vi "Set Current Range in Sweep.vi"(0 "VISA resource name":refnum<visa-resource-name>="GPIB0::24::INSTR", 5 "R":i32, 11 "error in (no error)":errorcluster) -> (4 "VISA resource name out":refnum<visa-resource-name>="GPIB0::24::INSTR", 15 "error out":errorcluster)   [LabVIEW 2010]
uses:
  <instrlib>/Keithley 2400/Keithley 24XX.lvlib
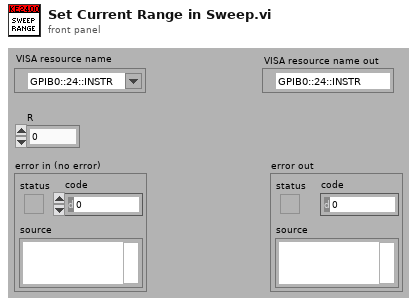
[diagram p1: front panel]
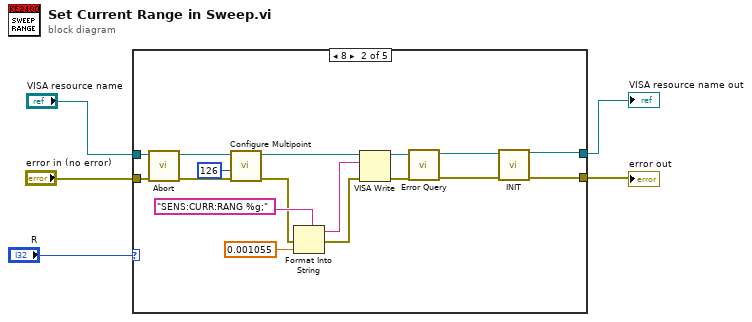
[diagram p0: block diagram]
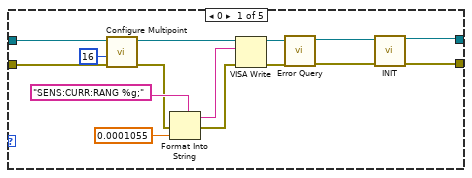
[diagram p2: hidden frame]
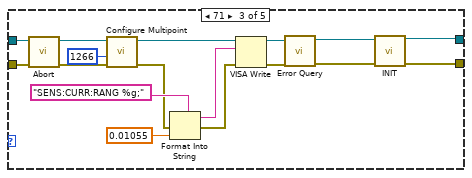
[diagram p3: hidden frame]
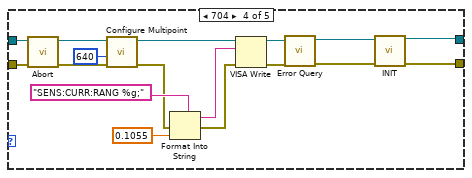
[diagram p4: hidden frame]
diagram:
  n1 = case shown="8" "R" {
    tunnel: [w15 w32 w49 w66 w73] -> w5
    tunnel: [w17 w34 w51 w68 w72] -> w4
    tunnel: "VISA resource name" -> [w10 w22 w39 w56 w73]
    tunnel: "error in (no error)" -> [w9 w27 w44 w61 w72]
    frame 0 {
      n2 = call <instrlib>:"Configure Multipoint.vi"("error in (no error)"=w9, "Trigger Count (1)"=16, "VISA resource name"=w10) -> ("error out"=w8:errorcluster, "VISA resource name out"=w7:refnum<visa-resource-name>)  [unwired: 7 in]
      n3 = Format Into String(format string="SENS:CURR:RANG %g;" ("Manual Range"), error in=w8, 0.0001055 ("R 2")) -> (resulting string=w12:string, error out=w11:errorcluster)  [unwired: 1 in]
      n4 = VISA Write(VISA resource name=w7, write buffer=w12, error in (no error)=w11) -> (VISA resource name out=w19:refnum<visa-resource-name>, error out=w18:errorcluster)  [unwired: 1 out]
      n5 = call <instrlib>:"Error Query.vi"("error in (no error)"=w18, "VISA resource name"=w19) -> ("error out"=w20:errorcluster, "VISA resource name out"=w16:refnum<visa-resource-name>)  [unwired: 6 in, 2 out]
      n6 = call "INIT.vi"("VISA resource name"=w16, "error in (no error)"=w20) -> ("VISA resource name out"=w15:refnum<visa-resource-name>, "error out"=w17:errorcluster)  [unwired: 12 in]
    }
    frame 8 {
      n7 = call <instrlib>:"Abort.vi"("error in (no error)"=w27, "VISA resource name"=w22) -> ("error out"=w23:errorcluster, "VISA resource name out"=w21:refnum<visa-resource-name>)  [unwired: 8 in]
      n8 = call <instrlib>:"Configure Multipoint.vi"("error in (no error)"=w23, "Trigger Count (1)"=126, "VISA resource name"=w21) -> ("error out"=w26:errorcluster, "VISA resource name out"=w25:refnum<visa-resource-name>)  [unwired: 7 in]
      n9 = Format Into String(format string="SENS:CURR:RANG %g;" ("Manual Range"), error in=w26, 0.001055 ("R 2")) -> (resulting string=w29:string, error out=w28:errorcluster)  [unwired: 1 in]
      n10 = VISA Write(VISA resource name=w25, write buffer=w29, error in (no error)=w28) -> (VISA resource name out=w36:refnum<visa-resource-name>, error out=w35:errorcluster)  [unwired: 1 out]
      n11 = call <instrlib>:"Error Query.vi"("error in (no error)"=w35, "VISA resource name"=w36) -> ("error out"=w37:errorcluster, "VISA resource name out"=w33:refnum<visa-resource-name>)  [unwired: 6 in, 2 out]
      n12 = call "INIT.vi"("VISA resource name"=w33, "error in (no error)"=w37) -> ("VISA resource name out"=w32:refnum<visa-resource-name>, "error out"=w34:errorcluster)  [unwired: 12 in]
    }
    frame 71 {
      n13 = call <instrlib>:"Abort.vi"("error in (no error)"=w44, "VISA resource name"=w39) -> ("error out"=w40:errorcluster, "VISA resource name out"=w38:refnum<visa-resource-name>)  [unwired: 8 in]
      n14 = call <instrlib>:"Configure Multipoint.vi"("error in (no error)"=w40, "Trigger Count (1)"=1266, "VISA resource name"=w38) -> ("error out"=w43:errorcluster, "VISA resource name out"=w42:refnum<visa-resource-name>)  [unwired: 7 in]
      n15 = Format Into String(format string="SENS:CURR:RANG %g;" ("Manual Range"), error in=w43, 0.01055 ("R 2")) -> (resulting string=w46:string, error out=w45:errorcluster)  [unwired: 1 in]
      n16 = VISA Write(VISA resource name=w42, write buffer=w46, error in (no error)=w45) -> (VISA resource name out=w53:refnum<visa-resource-name>, error out=w52:errorcluster)  [unwired: 1 out]
      n17 = call <instrlib>:"Error Query.vi"("error in (no error)"=w52, "VISA resource name"=w53) -> ("error out"=w54:errorcluster, "VISA resource name out"=w50:refnum<visa-resource-name>)  [unwired: 6 in, 2 out]
      n18 = call "INIT.vi"("VISA resource name"=w50, "error in (no error)"=w54) -> ("VISA resource name out"=w49:refnum<visa-resource-name>, "error out"=w51:errorcluster)  [unwired: 12 in]
    }
    frame 704 {
      n19 = call <instrlib>:"Abort.vi"("error in (no error)"=w61, "VISA resource name"=w56) -> ("error out"=w57:errorcluster, "VISA resource name out"=w55:refnum<visa-resource-name>)  [unwired: 8 in]
      n20 = call <instrlib>:"Configure Multipoint.vi"("error in (no error)"=w57, "Trigger Count (1)"=640, "VISA resource name"=w55) -> ("error out"=w60:errorcluster, "VISA resource name out"=w59:refnum<visa-resource-name>)  [unwired: 7 in]
      n21 = Format Into String(format string="SENS:CURR:RANG %g;" ("Manual Range"), error in=w60, 0.1055 ("R 2")) -> (resulting string=w63:string, error out=w62:errorcluster)  [unwired: 1 in]
      n22 = VISA Write(VISA resource name=w59, write buffer=w63, error in (no error)=w62) -> (VISA resource name out=w70:refnum<visa-resource-name>, error out=w69:errorcluster)  [unwired: 1 out]
      n23 = call <instrlib>:"Error Query.vi"("error in (no error)"=w69, "VISA resource name"=w70) -> ("error out"=w71:errorcluster, "VISA resource name out"=w67:refnum<visa-resource-name>)  [unwired: 6 in, 2 out]
      n24 = call "INIT.vi"("VISA resource name"=w67, "error in (no error)"=w71) -> ("VISA resource name out"=w66:refnum<visa-resource-name>, "error out"=w68:errorcluster)  [unwired: 12 in]
    }
    frame 1, Default {
    }
  }
  "VISA resource name out" <- w5
  "error out" <- w4
